vi "BAP3P.vi"(5 "Header Comments":string="This is a C(T) experiment being done in Physics 350.\r\nIt records the decay response of an RC circuit where the capacitance is a strong function of temperature.", 7 "Temperature Control Parameters":T1={"Start Temp"=30.0, "Temp Step"=5.0, "End Temp"=80.0} {"End Temp" format="%.2f"; "Temp Step" format="%.2f"; "Start Temp" format="%.2f"}, 9 "Timing Control Parameters":T2={"N cycles for averaging"=10, "N points per measurment"=1000, "Measurment time interval"=2e-05} {"Measurment time interval" format="%.2e"}, 11 "error in":errorcluster) -> (4 "Auto Launch Data Viewer at End":bool=TRUE, 6 "data file path out":path, 8 "Temp Array":dbl[](array[numeric]), 10 "Timing Control Parameters out":T2={"N cycles for averaging"=10, "N points per measurment"=1000, "Measurment time interval"=2e-05} {"Measurment time interval" format="%.2e"}, 15 "error out":errorcluster)   [LabVIEW 2014]
doc: "BAP3B\n\nInputs Temperature and Timing Control Parameters from front panel or from a file and displays header comments, file header with labels for corresponding data, and gives the option of creating a data before exiting. The Proeed and Auto Launch Viewer are indicators utilized in upcoming projects.\n\nError input and output is applied. \n\nSubVis Modified:\nTemp Gen Aray BAP3B\nDate Time Str Converter BAP3P\n\nBeverly Abadines\nPHY 350\nBAP3B"
uses:
  typedefs/time control params.ctl
  typedefs/temp control params.ctl
panel:
  out "File Header":string="This is a C(T) experiment being done in Physics 350.\r\nIt records the decay response of an RC circuit where the capacitance is a strong function of temperature.\n\n2/14/2007\n1:53 PM\r\n\r\nStart temp = 30.0\r\nTemp step = 10.0\r\nEnd temp = 80.0\r\nNum temps = 6\r\nNum avg cycles = 10\r\nNum points per meas = 1000\r\nMeas time interval = 2.00E-5\n\nDDD\n\n"
  out "Proceed":bool
  in  "exit":bool
  in  "create file and proceed":bool
  in  "reload parameters 2":bool
  in  "Auto Launch Data Viewer at End":bool=TRUE
  out "Warning":bool=TRUE
  out "N temps 2":i32=6
  # "Beverly Abadines\nPhys 350"
  # "BAP3P"
  # "P350 C(T) Experimental Initialization"
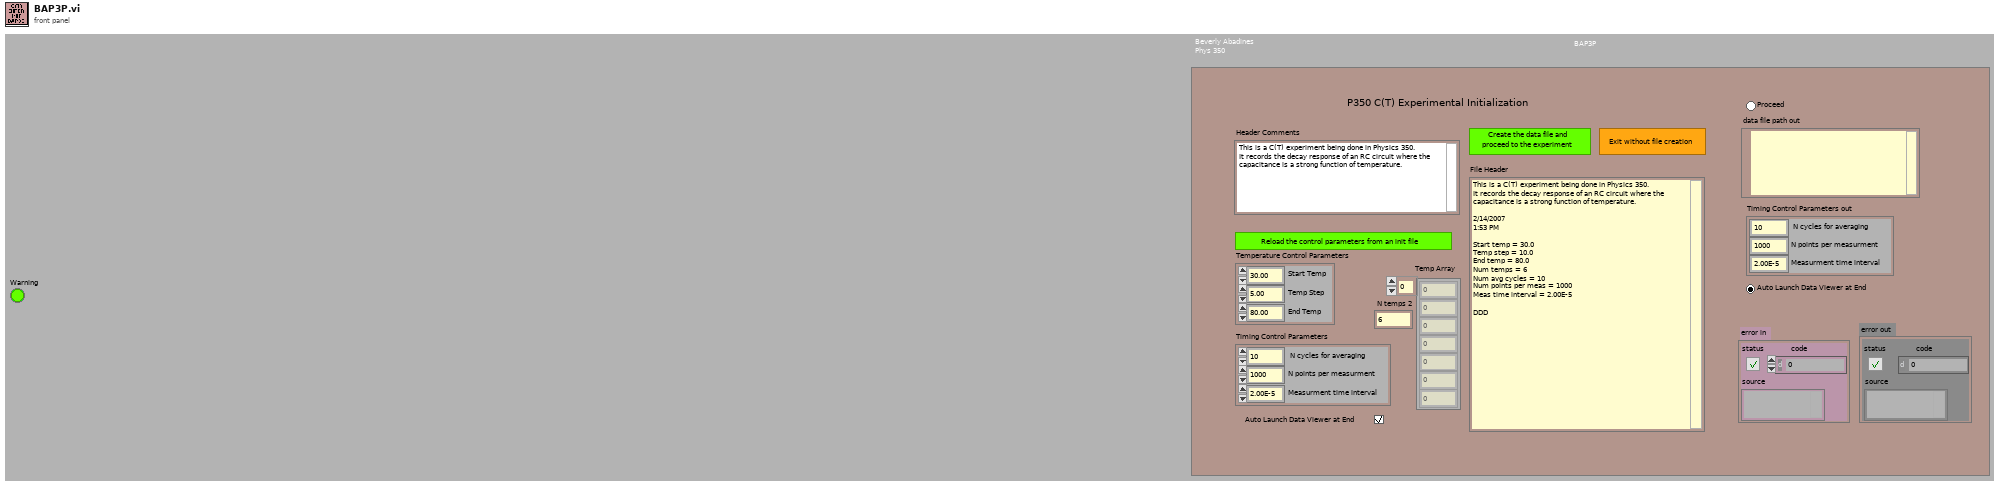
[diagram p1: front panel]
types:
  T1 = typedef "temp control params.ctl" = cluster{"Start Temp":dbl, "Temp Step":dbl, "End Temp":dbl}
  T2 = typedef "time control params.ctl" = cluster{"N cycles for averaging":i32, "N points per measurment":i32, "Measurment time interval":dbl}
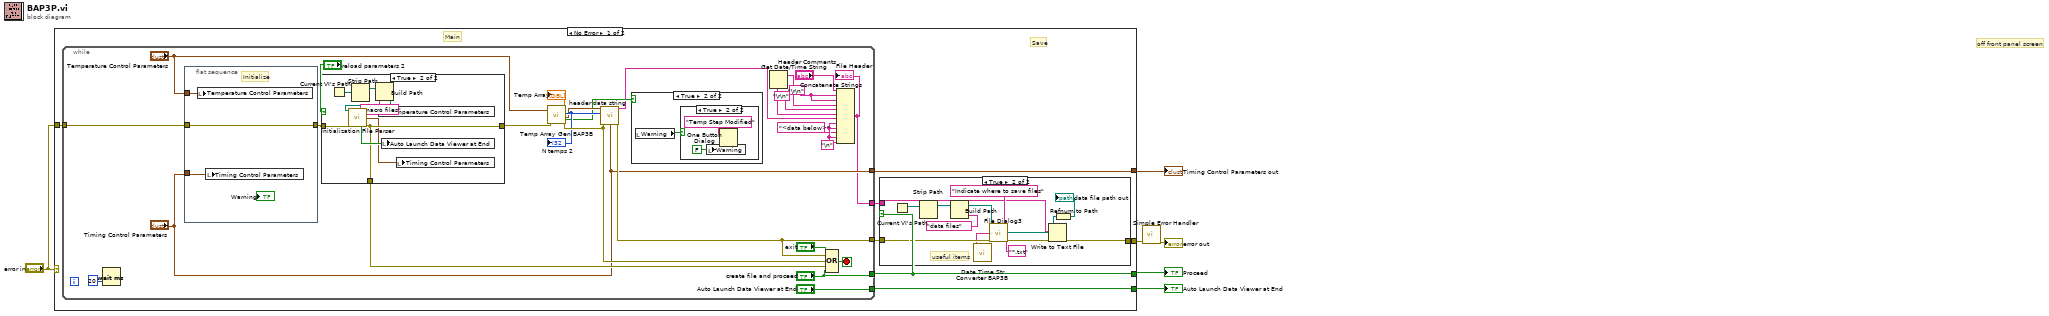
[diagram p0: block diagram]
diagram:
  # "useful items"
  # "off front panel screen"
  n1 = case shown="No Error" "error in" {
    selector: "error in" -> [_ w70]
    tunnel: "error in" -> [w12 _]
    tunnel: [w7 w70] -> w6
    tunnel: [w8 _] -> w2
    tunnel: [w13 _] -> w3
    tunnel: [w11 _] -> w1
    frame No Error {
      # "Save"
      # "Main"
      n2 = while {
        tunnel: [w42] -> w9
        tunnel: [w28] -> w10
        tunnel: ["create file and proceed"] -> w8
        tunnel: ["Auto Launch Data Viewer at End"] -> w13
        tunnel: w12 -> [w47]
        tunnel: ["Timing Control Parameters"] -> w11
        stop <- w52 stop-if-true
        w30 = "\r\n" ("string")
        w36 = "\n"
        n3 = Wait (ms)(milliseconds to wait=u32 20) -> ()  [unwired: 1 out]
        n4 = flat-sequence {
          tunnel: "Timing Control Parameters" -> [w60]
          tunnel: "Temperature Control Parameters" -> [w59]
          tunnel: w47 -> [w58]
          tunnel: [w58] -> w46
          frame #0 {
            # "Initialize"
            n5 = local write "Temperature Control Parameters"(w59) -> ()
            n6 = local write "Timing Control Parameters"(w60) -> ()
          }
        }
        n7 = case shown="True" "reload parameters 2" {
          tunnel: [_ w68] -> w44
          tunnel: [_ w68] -> w50
          tunnel: w46 -> [_ w65]
          frame False {
          }
          frame True {
            n8 = Current VI's Path() -> (path=w63:path)
            n9 = Strip Path(path=w63) -> (stripped path=w64:path)  [unwired: 1 out]
            n10 = Build Path(base path=w64, name or relative path="macro files") -> (appended path=w61:path)
            n11 = call "Initialization File Parser.vi"("path in"=w61, "error in"=w65) -> ("Auto Launch Data Viewer at End"=w69:bool, "temp control parameters"=w66:T1, "time control parameters"=w67:T2, "error out"=w68:errorcluster)  [unwired: 9 in, 1 out]
            n12 = local write "Temperature Control Parameters"(w66) -> ()
            n13 = local write "Auto Launch Data Viewer at End"(w69) -> ()
            n14 = local write "Timing Control Parameters"(w67) -> ()
          }
        }
        n15 = call "Temp Array Gen BAP3B.vi"("error in (no error)"=w44, "Temperature Control Parameters"="Temperature Control Parameters") -> ("error out"=w43:errorcluster, "Temperature Control Parameters Out"=w38:T1, "N Temps"=w41:i32, "Temp Array"=→"Temp Array":dbl[], "Warning"=w37:bool)  [unwired: 5 in]
        "N temps 2" <- w41
        n16 = call "header data string.vi"("Temperature Control Parameters"=w38, "N temps"=w41, "error in (no error)"=w43, "Timing Control Parameters"="Timing Control Parameters") -> ("Header string component"=w29:string, "error out"=w42:errorcluster)  [unwired: 10 in]
        n17 = case shown="True" w37 {
          frame False {
          }
          frame True {
            n18 = local read "Warning"() -> (w55:bool)
            n19 = case shown="True" w55 {
              frame False {
              }
              frame True {
                n20 = local write "Warning"(FALSE ("Warning")) -> ()
                n21 = One Button Dialog(message="Temp Step Modified") -> ()  [unwired: 1 in, 1 out]
              }
            }
          }
        }
        n22 = Get Date/Time String() -> (date string=w34:string, time string=w32:string)  [unwired: 1 in, 2 out]
        n23 = Compound Arithmetic op=OR("exit", w42, w43, w50, "create file and proceed") -> (w52:bool)
        n24 = Concatenate Strings("Header Comments", w30, w30, w34, "\r\n" ("string"), w32, w29, w36, w36, "<data below>", w36, w36) -> (w28:string)
        "File Header" <- w28
      }
      n25 = case shown="True" w8 {
        tunnel: [w14 w18] -> w7
        tunnel: w9 -> [w14 w26]
        tunnel: w10 -> [_ w17]
        frame False {
        }
        frame True {
          n26 = Current VI's Path() -> (path=w20:path)
          n27 = Strip Path(path=w20) -> (stripped path=w22:path)  [unwired: 1 out]
          n28 = Build Path(base path=w22, name or relative path="data files") -> (appended path=w23:path)
          n29 = call "Date Time Str Converter BAP3B.vi"() -> ("String Output"=w19:string)  [unwired: 11 in]
          n30 = call "File Dialog3"("start path"=w23, "prompt"="Indicate where to save files" ("prompt (Choose or enter file path)"), "default name"=w19, "pattern (all files)"="*.txt" ("pattern")) -> ("selected path"=w21:path)  [unwired: 8 in, 3 out]
          n31 = Write to Text File(file (use dialog)=w21, text=w17, error in=w26) -> (refnum out=w27:refnum<file>, error out=w18:errorcluster)  [unwired: 1 in, 1 out]
          n32 = Refnum to Path(1:w27) -> (0:→"data file path out":path)
        }
      }
    }
    frame Error {
    }
  }
  "Timing Control Parameters out" <- w1
  "Auto Launch Data Viewer at End" <- w3
  "Proceed" <- w2
  n33 = call <vilib>:"Simple Error Handler.vi"("error in (no error)"=w6) -> ("error out"=→"error out":errorcluster)  [unwired: 4 in, 4 out]
